vi "Scan Bracketed String.vi"(5 "Include Brackets (F)":bool, 7 "Offset (0)":i32, 9 "End":string, 10 "Start":string, 11 "String":string) -> (1 "Empty Scan":bool, 2 "Nested":bool, 3 "Substring":string)   [LabVIEW 2013, in "LV JSON.lvlib"]
doc: "Search String for bracketed string (string with Start string before it and End string at after it) such that no nested bracketed strings are broken. Set Include Brackets to True to inclue Start and End strings in Substring output.\n\nExample:\nString = {\"Array\":[[1,2,3],[4,5,6],[7,8,9]]}\nStart = [\nEnd = ]\nOffset (0) = 0\nInclude Brackets (F) = False\nSubstring = [1,2,3],[4,5,6],[7,8,9]"
uses:
  LV JSON.lvlib
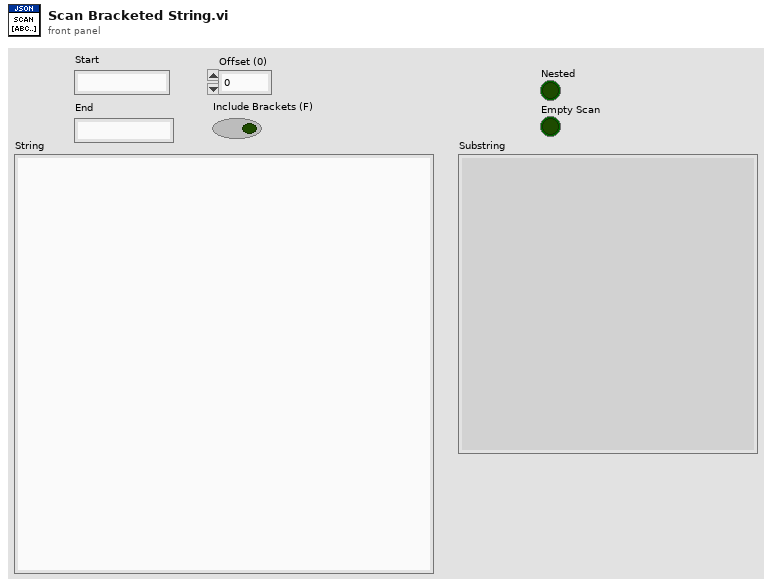
[diagram p1: front panel]
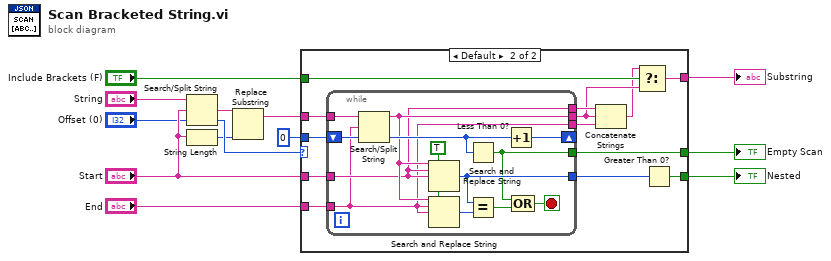
[diagram p0: block diagram]
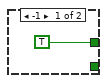
[diagram p2: hidden frame]
diagram:
  n1 = Search/Split String(string="String", search string/char (-)="Start", offset (0)="Offset (0)") -> (match + rest of string=w4:string, offset of match=w5:i32)  [unwired: 1 out]
  n2 = String Length(string="Start") -> (length=w3:i32)
  n3 = Replace Substring(2:w3, 5:w4) -> (1:w2:string)  [unwired: 2 in, 1 out]
  n4 = case shown="Default" w5 {
    tunnel: "End" -> [_ w27]
    tunnel: w2 -> [_ w25]
    tunnel: 0 ("offset past match") -> [_ w24]
    tunnel: "Start" -> [_ w23]
    tunnel: [_ w16] -> w9
    tunnel: "Include Brackets (F)" -> [_ w21]
    tunnel: [_ w22] -> w7
    tunnel: [TRUE w15] -> w1
    frame -1 {
    }
    frame Default {
      n5 = while {
        tunnel: w25 -> [w36]
        shift-right: [w33] -> _
        shift-left: w24 -> [w35]
        tunnel: [w31] -> w18
        tunnel: w27 -> [w29]
        tunnel: w23 -> [w30]
        tunnel: [w39] -> w26
        tunnel: [w30] -> w20
        tunnel: [w29] -> w19
        tunnel: [w28] -> w15
        stop <- w37 stop-if-true
        w32 = TRUE ("replace all? (F)")
        n6 = Search/Split String(string=w36, search string/char (-)=w29, offset (0)=w35) -> (substring before match=w31:string, offset of match=w34:i32)  [unwired: 1 out]
        n7 = Search and Replace String(replace all?=w32, input string=w31, search string=w30, replace string=w30) -> (number of replacements=w39:i32)  [unwired: 4 in, 3 out]
        n8 = Search and Replace String(replace all?=w32, input string=w31, search string=w29, replace string=w29) -> (number of replacements=w40:i32)  [unwired: 4 in, 3 out]
        n9 = Less Than 0?(x=w34) -> (x < 0?=w28:bool)
        n10 = Equal?(x=w39, y=w40) -> (x = y?=w38:bool)
        n11 = Increment(x=w34) -> (x+1=w33:i32)
        n12 = Compound Arithmetic op=OR(w28, w38) -> (w37:bool)
      }
      n13 = Concatenate Strings(w20, w18, w19) -> (w17:string)
      n14 = Select(t=w17, s=w21, f=w18) -> (s? t:f=w16:string)
      n15 = Greater Than 0?(x=w26) -> (x > 0?=w22:bool)
    }
  }
  "Substring" <- w9
  "Nested" <- w7
  "Empty Scan" <- w1
